vi "Save Log File.vi"(8 "error in (no error)":errorcluster, 9 "Path":path, 10 "Logged Data":dbl[][](array[numeric]), 11 "VISA resource name":refnum<visa-resource-name>) -> (0 "error out":errorcluster, 3 "VISA resource name out":refnum<visa-resource-name>)   [LabVIEW 2013, in "Watts Up Series.lvlib"]
uses:
  <instrlib>/Watts Up Series/Watts Up Series.lvlib
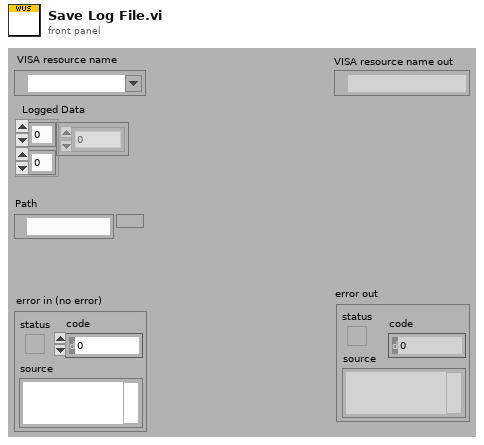
[diagram p1: front panel]
types:
  T1 = enum16{"open", "replace", "create", "open or create", "replace or create", "replace or create with confirmation"}
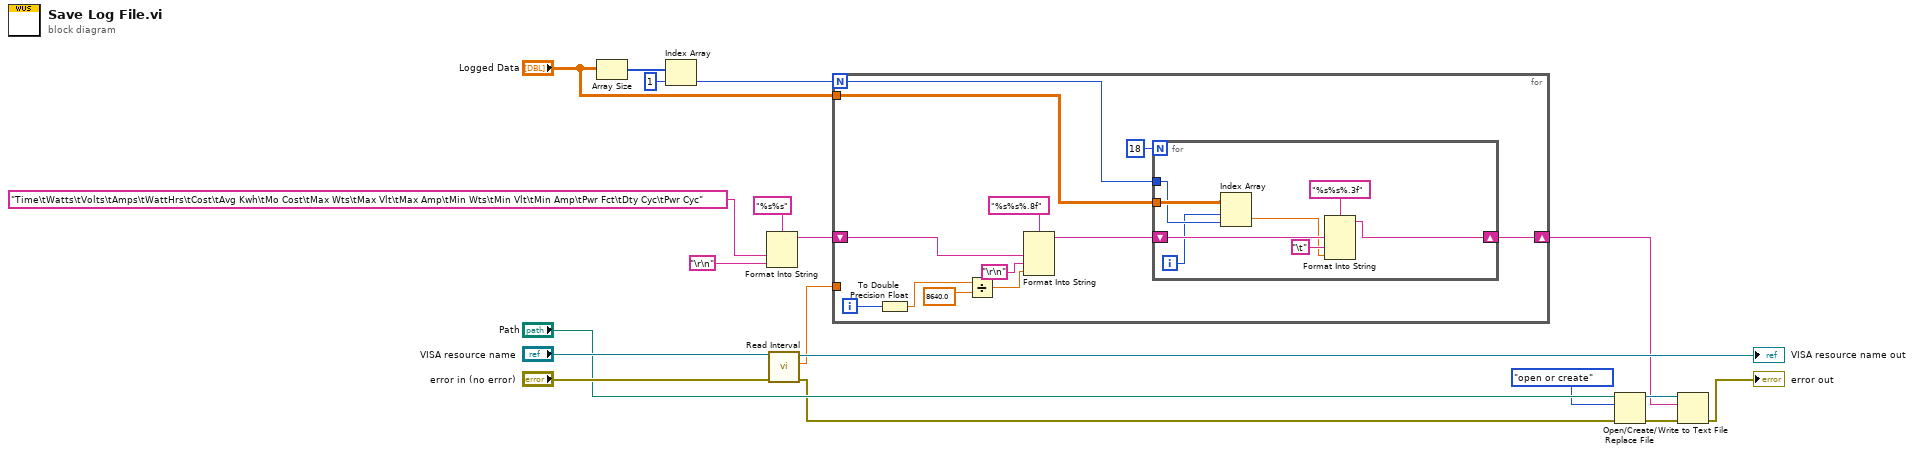
[diagram p0: block diagram]
diagram:
  n1 = Array Size(array="Logged Data") -> (size(s)=w16:i32[])
  n2 = Index Array(array=w16, index=1) -> (element=w2:i32)
  n3 = Format Into String(format string="%s%s", "Time\tWatts\tVolts\tAmps\tWattHrs\tCost\tAvg Kwh\tMo Cost\tMax Wts\tMax Vlt\tMax Amp\tMin Wts\tMin Vlt\tMin Amp\tPwr Fct\tDty Cyc\tPwr Cyc" ("text"), "\r\n") -> (resulting string=w12:string)  [unwired: 2 in, 1 out]
  n4 = call <instrlib>:"Read Interval.vi"("error in (no error)"="error in (no error)", "VISA resource name"="VISA resource name") -> ("error out"=w8:errorcluster, "Record Interval"=w13:dbl, "VISA resource name out"=→"VISA resource name out":refnum<visa-resource-name>)  [unwired: 7 in]
  n5 = for {
    N: w2 -> [w23]
    tunnel: w13 -> [_]
    shift-right: [w20] -> w4
    shift-left: w12 -> [w30]
    tunnel: "Logged Data" -> [w22]
    i -> [w28]
    n6 = To Double Precision Float(number=w28) -> (double precision float=w27:dbl)
    n7 = Divide(x=w27, y=8640.0) -> (x/y=w25:dbl)
    n8 = Format Into String(format string="%s%s%.8f", w30, "\r\n", w25) -> (resulting string=w21:string)  [unwired: 2 in, 1 out]
    n9 = for {
      N: 18 -> [_]
      tunnel: w23 -> [w38]
      tunnel: w22 -> [w39]
      shift-right: [w33] -> w20
      shift-left: w21 -> [w37]
      i -> [w32]
      n10 = Index Array(array=w39, index (row)=w32, index (col)=w38) -> (element=w34:dbl)
      n11 = Format Into String(format string="%s%s%.3f", w37, "\t", w34) -> (resulting string=w33:string)  [unwired: 2 in, 1 out]
    }
  }
  n12 = Open/Create/Replace File(file path (use dialog)="Path", error in=w8, operation (0:open)=T1."open or create") -> (refnum out=w5:refnum<file>, error out=w6:errorcluster)  [unwired: 3 in, 1 out]
  n13 = Write to Text File(file (use dialog)=w5, text=w4, error in=w6) -> (error out=→"error out":errorcluster)  [unwired: 1 in, 2 out]
